vi "atiMatrixMult.vi"(2 "error in (no error)":errorcluster, 3 "Voltages":dbl[](array[numeric]), 4 "Calibration Matrix":dbl[][](array[numeric])) -> (0 "error out":errorcluster, 1 "F/T Data":dbl[](array[numeric]))   [LabVIEW 2012]
doc: "Takes a calibration matrix and voltage vector and mutliplies them to get resolved force/torque data."
uses:
  <vilib>/Analysis/baseanly.llb/A x Vector.vi
  <vilib>/Analysis/NI_AALBase.lvlib
  <vilib>/Analysis/NI_AALPro.lvlib
  <vilib>/Analysis/coordinate.llb/2D Cartesian Coordinate Rotation (Scalar).vi
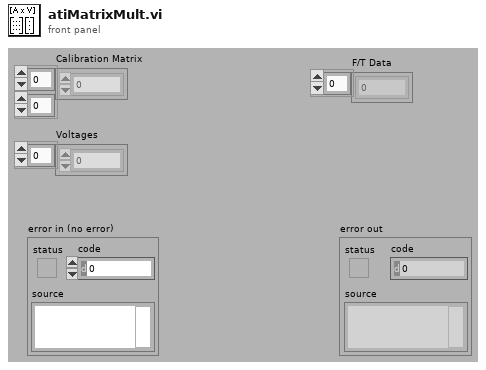
[diagram p1: front panel]
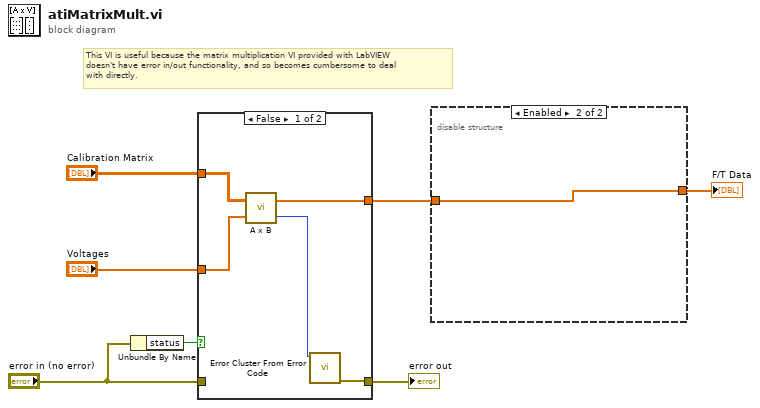
[diagram p0: block diagram]
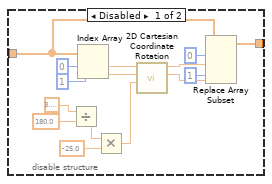
[diagram p2: hidden frame]
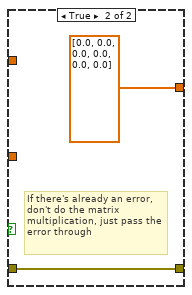
[diagram p3: hidden frame]
diagram:
  # "This VI is useful because the matrix multiplication VI provided with LabVIEW\ndoesn't have error in/out functionality, and so becomes cumbersome to deal\nwith directly."
  n1 = Unbundle By Name("error in (no error)") -> ("status"=w5:bool)
  n2 = case shown="False" w5 {
    tunnel: [w9 w14] -> w7
    tunnel: "error in (no error)" -> [_ w14]
    tunnel: "Calibration Matrix" -> [w12 _]
    tunnel: "Voltages" -> [w11 _]
    tunnel: [w8 dbl[] [0.0, 0.0, 0.0, 0.0, 0.0, 0.0]] -> w2
    frame False {
      n3 = call-poly <vilib>:"A x B.vi"("Vector"=w11, "A"=w12) -> ("error"=w10:i32, "A x Vector"=w8:dbl[])
      n4 = call <vilib>:"Error Cluster From Error Code.vi"("error code (0)"=w10) -> ("error out"=w9:errorcluster)  [unwired: 8 in]
    }
    frame True {
      # "If there's already an error, \ndon't do the matrix\nmultiplication, just pass the\nerror through"
    }
  }
  "error out" <- w7
  n5 = disable-structure shown="Enabled" {
    disable-tunnel: w2 -> [w20 w30]
    disable-tunnel: [w19 w30] -> w1
    frame Disabled {
      n6 = Divide(x=3.141592653589793, y=180.0) -> (x/y=w23:dbl)
      n7 = Index Array(array=w20, index #1=0 ("index"), index #2=1 ("index")) -> (element #1=w27:dbl, element #2=w26:dbl)
      n8 = Multiply(x=w23, y=-25.0) -> (x*y=w21:dbl)
      n9 = call-poly <vilib>:"2D Cartesian Coordinate Rotation.vi"("theta"=w21, "y"=w26, "x"=w27) -> ("y out"=w17:dbl, "x out"=w18:dbl)  [unwired: 6 in, 1 out]
      n10 = Replace Array Subset(array=w20, new element #1=w18, index #1=0 ("index"), new element #2=w17, index #2=1 ("index")) -> (w19:dbl[])
    }
    frame Enabled {
    }
  }
  "F/T Data" <- w1
